vi "Pfeiffer Vacuum Digiline Adjust.vi"(8 "error in (no error)":errorcluster, 9 "Digiline adjustment - Cluster":T1 {"Switch Filament HPT200" items=["Filament auto (default)", "Filament 1", "Filament 2"]; "Sensor Switch Mode" items=["switch", "trans_Lo", "trans_Hi"]; "Parameter" items=[" DeGas (on/off)  (for HPT only) ", " Sensor (on/off)", " Sensor Switch Mode", " Switch Filament (for HPT200 only)"]}, 10 "Adress of unit":u16=1 min=1 max=999 step=1, 11 "VISA session in":refnum<visa-resource-name>) -> (0 "error out":errorcluster, 3 "response (data)":string)   [LabVIEW 2016]
doc: "This VI is an example of how to use the Pfeiffer Vacuum subVIs programmatically. This VI first initializes the instrument, takes measurements, then closes the instrument."
uses:
  Public/DigiLine/DigiLine adjustment - Cluster.ctl
  Pfeiffer Vacuum.lvlib
panel:
  # "<-------          ------->     \n DeGas (on/off)   :       off                   on             \n Sensor (on/off)  :       off                   on"
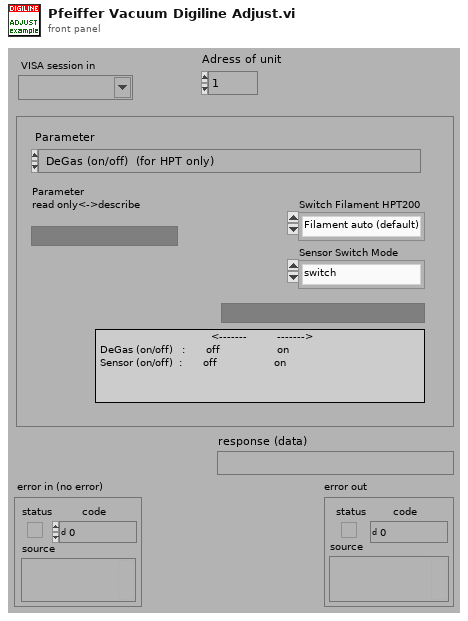
[diagram p1: front panel]
types:
  T1 = typedef "Pfeiffer Vacuum.lvlib/DigiLine adjustment - Cluster.ctl" = cluster{"Parameter":u16, "Parameter\nread only<->describe":bool, "off/on":bool, "Sensor Switch Mode":u16, "Switch Filament HPT200":u16}
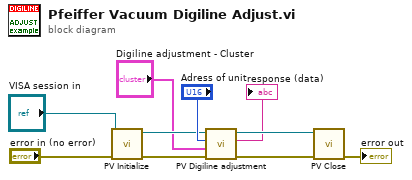
[diagram p0: block diagram]
diagram:
  n1 = call "PV Initialize.vi"("error in (no error)"="error in (no error)", "VISA session in"="VISA session in") -> ("error out"=w4:errorcluster, "VISA session out"=w3:refnum<visa-resource-name>)  [unwired: 8 in]
  n2 = call "PV Digiline adjustment.vi"("error in (no error)"=w4, "Digiline adjustment - Cluster"="Digiline adjustment - Cluster", "Adress of unit"="Adress of unit", "VISA session"=w3) -> ("error out"=w10:errorcluster, "response (data)"=→"response (data)":string, "dup VISA session"=w9:refnum<visa-resource-name>)  [unwired: 5 in]
  n3 = call "PV Close.vi"("VISA session"=w9, "error in (no error)"=w10) -> ("error out"=→"error out":errorcluster)  [unwired: 13 in]
